vi "Initialize.vi"(8 "error in (no error)":errorcluster, 9 "Channel":i32, 10 "VISA resource name":refnum<visa-resource-name>, 11 "VirtualPower in":refnum<class "VirtualPower.lvclass">) -> (0 "error out":errorcluster, 3 "VirtualPower out":refnum<class "VirtualPower.lvclass">)   [LabVIEW 2020, in "PowerControl.lvlib" / "VirtualPower.lvclass"]
uses:
  VirtualPower.lvclass
  VirtualPower.lvclass/VirtualPower.ctl
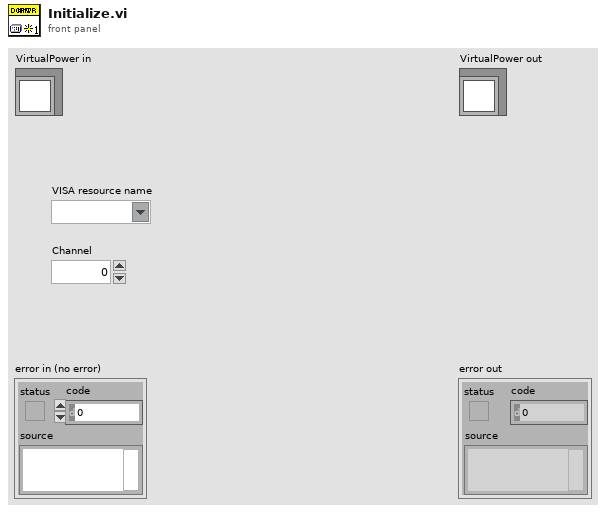
[diagram p1: front panel]
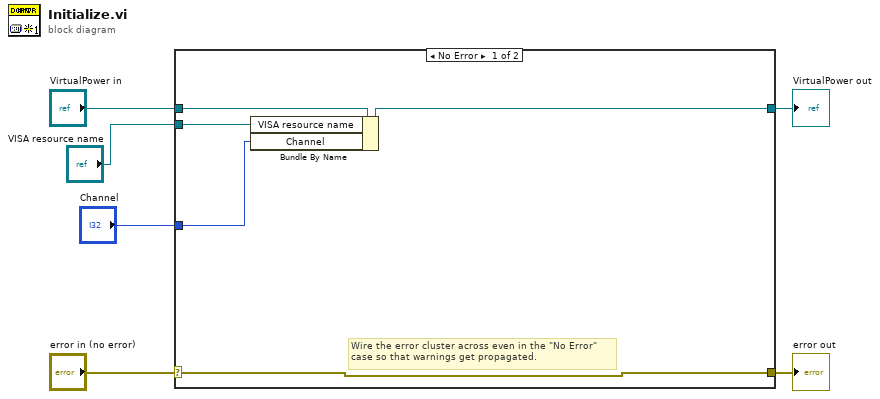
[diagram p0: block diagram]
diagram:
  n1 = case shown="No Error" "error in (no error)" {
    selector: "error in (no error)" -> [w7 w13]
    tunnel: [w7 w13] -> w5
    tunnel: [w10 w12] -> w3
    tunnel: "VirtualPower in" -> [w11 w12]
    tunnel: "VISA resource name" -> [w8 _]
    tunnel: "Channel" -> [w9 _]
    frame No Error {
      # "Wire the error cluster across even in the \"No Error\"\ncase so that warnings get propagated."
      n2 = Bundle By Name(cluster=w11, "VISA resource name"=w8, "Channel"=w9) -> (w10:refnum<class "VirtualPower.lvclass">)
    }
    frame Error {
    }
  }
  "error out" <- w5
  "VirtualPower out" <- w3
